vi "外观 2.vi"(0 "Data In":T5 caption="数据输入" format="%04x", 2 "Display State In":T3 caption="显示状态输入", 3 "Container State":T4 caption="容器状态") -> (6 "Data Out":T5 caption="数据输出" format="%04x", 7 "Display State Out":T3 caption="显示状态输出", 8 "Action":T2 caption="动作")   [LabVIEW 2016, in "总磷氨氮调试.xctl"]
uses:
  <vilib>/_xctls/Container State.ctl
  <vilib>/_xctls/Action.ctl
  <vilib>/_xctls/XControlSupport.lvlib
panel:
  out "选项卡控件":enum32{"选项卡 1", "选项卡 2"}(tab)
  in  "V9-2":bool
  in  "V9-1":bool
  in  "阀口选择":T1(radio)
  in  "阀口":enum32{"未选择", "V1开", "V1关", "V2开", "V2关"}(radio)
  in  "蠕动泵":enum32{"未选择", "P1", "P2"}(radio)
  in  "灯":enum32{"未选择", "520", "660", "加热恒温", "氙灯/紫灯"}(radio)
  in  "ADC值":enum32{"未选择", "ADC0", "降温温度", "消解温度", "光谱/ADC1"}(radio)
  in  "总磷总氮启动项目输入":enum32{"功能1", "功能2"}(ring)
  in  "功能选择":enum32{"等待", "复位", "注入", "注出"}(radio)=enum."注入"
  in  "数值":i16=4000
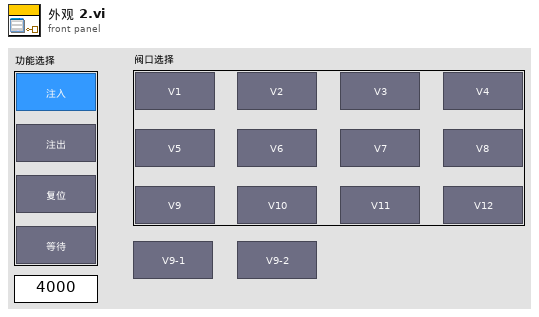
[diagram p1: front panel]
types:
  T1 = enum32{"未选择", "V1", "V2", "V3", "V4", "V5", "V6", "V7", "V8", "V9", "V10", "V11", "V12"}
  T2 = typedef "XControlSupport.lvlib/Action.ctl" = cluster{"Data Changed?":bool, "State Changed?":bool, "Action Name":string}
  T3 = typedef "总磷氨氮调试.xctl/状态 2.ctl" = cluster{"Numeric":dbl}
  T4 = typedef "XControlSupport.lvlib/Container State.ctl" = cluster{"Indicator?":bool, "Run Mode?":bool, " Refnum":refnum<vi>}
  T5 = typedef "总磷氨氮调试.xctl/数据 2.ctl" = u16[]
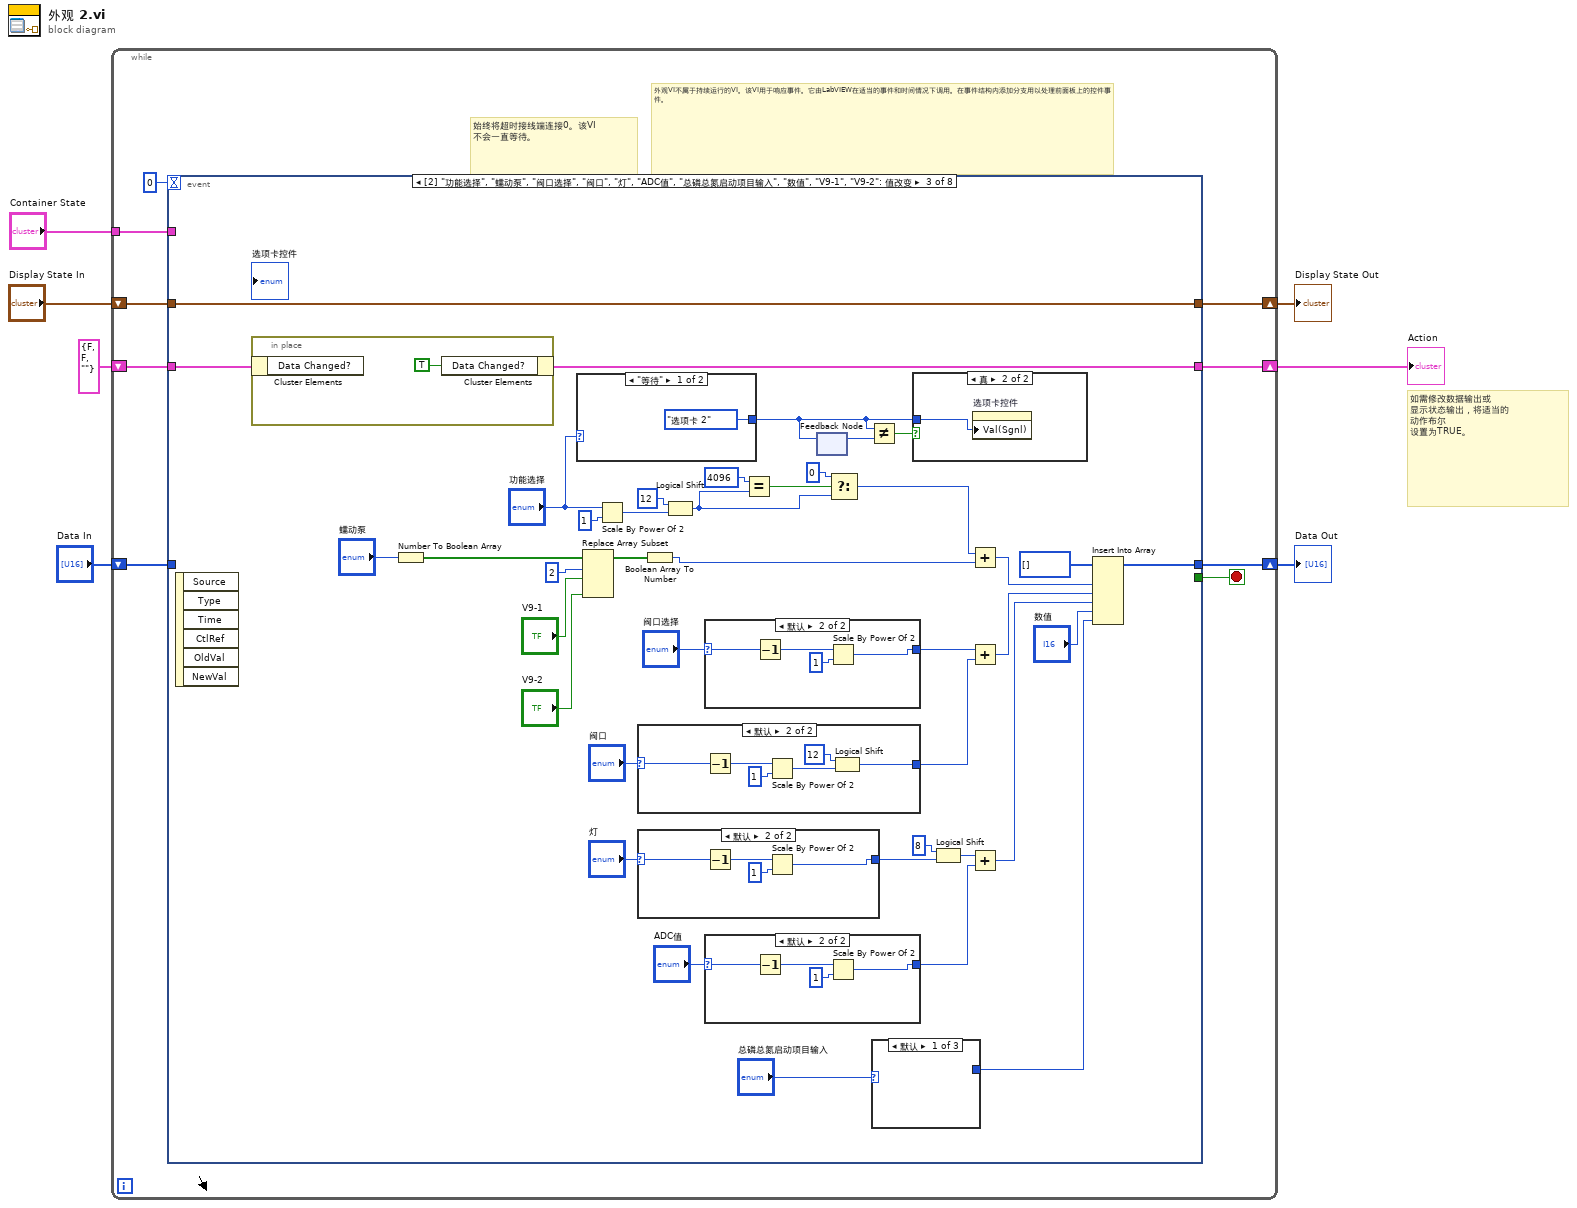
[diagram p0: block diagram]
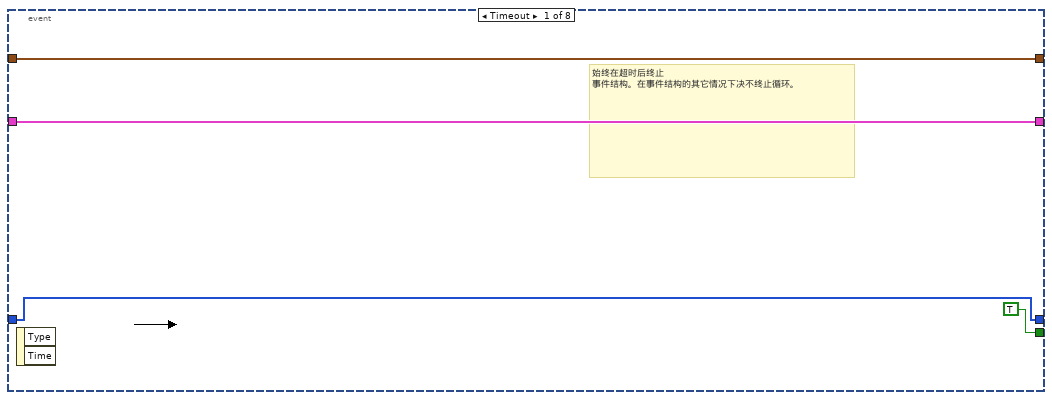
[diagram p2: hidden frame]
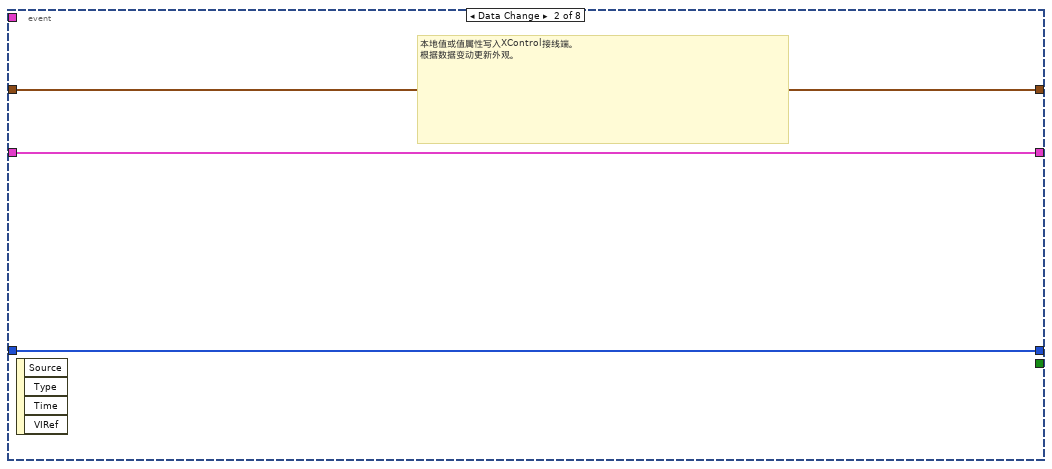
[diagram p3: hidden frame]
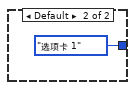
[diagram p5: hidden frame]
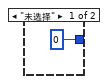
[diagram p6: hidden frame]
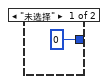
[diagram p7: hidden frame]
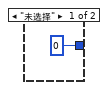
[diagram p8: hidden frame]
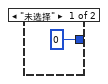
[diagram p9: hidden frame]
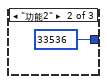
[diagram p10: hidden frame]
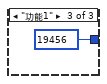
[diagram p11: hidden frame]
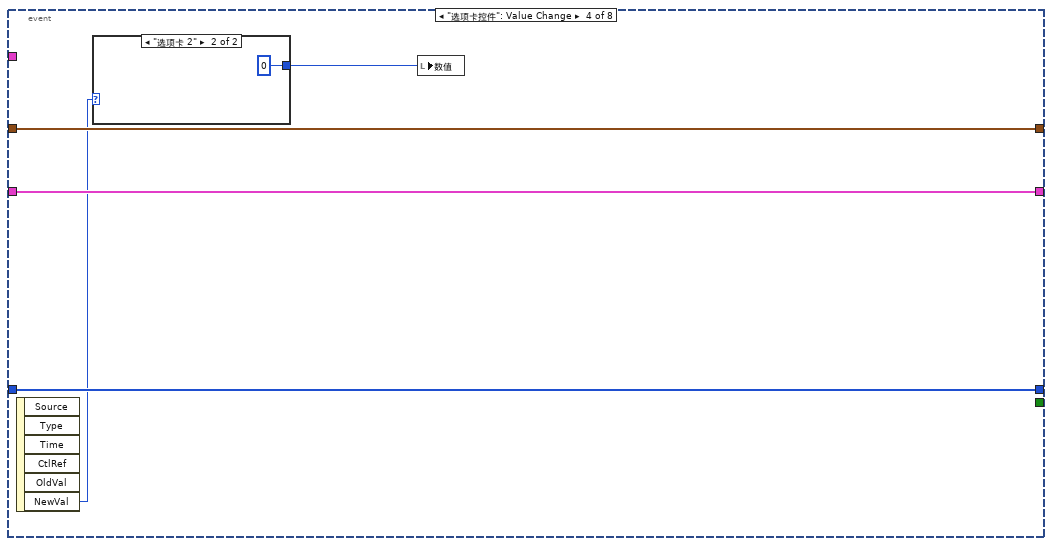
[diagram p12: hidden frame]
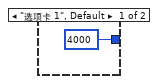
[diagram p13: hidden frame]
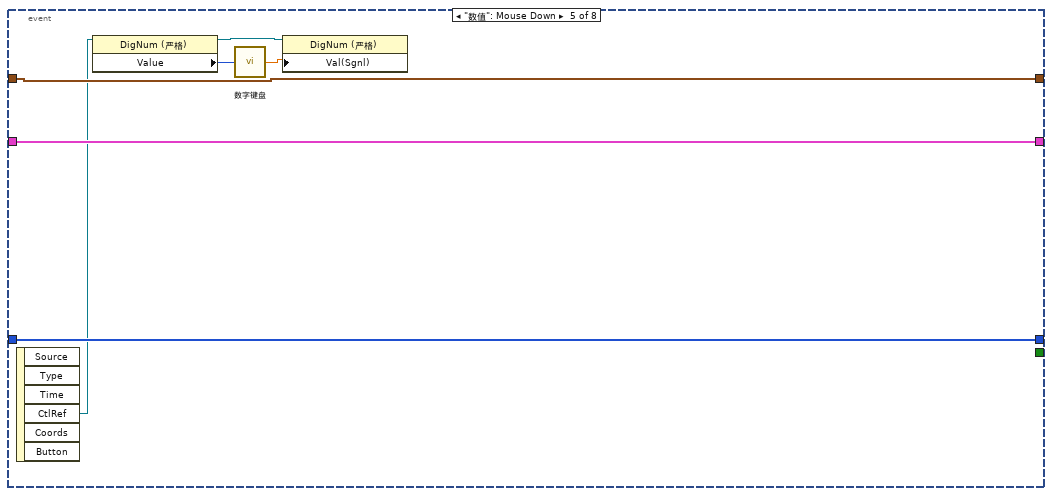
[diagram p14: hidden frame]
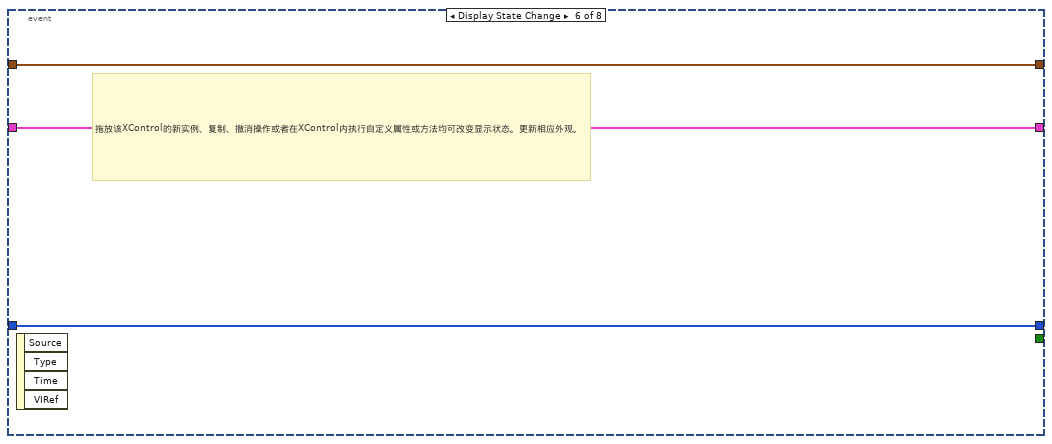
[diagram p15: hidden frame]
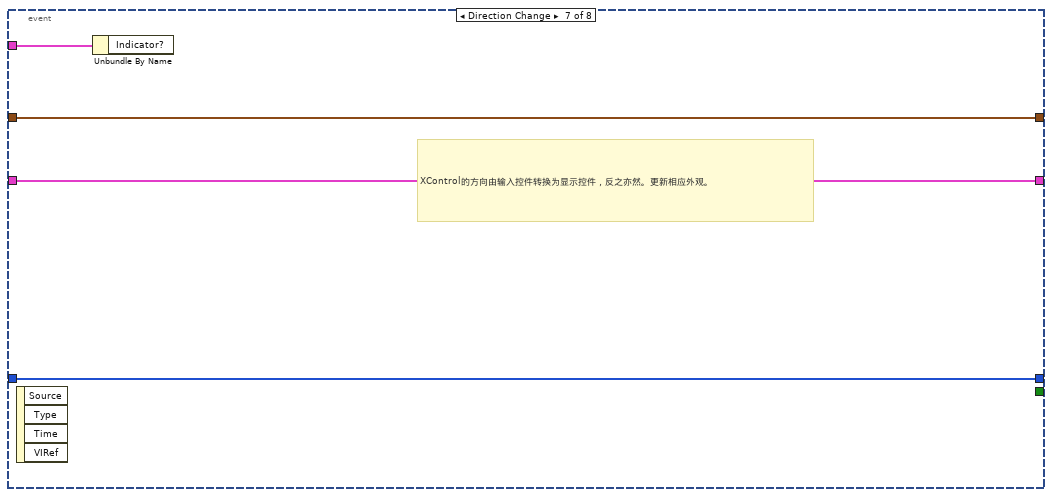
[diagram p16: hidden frame]
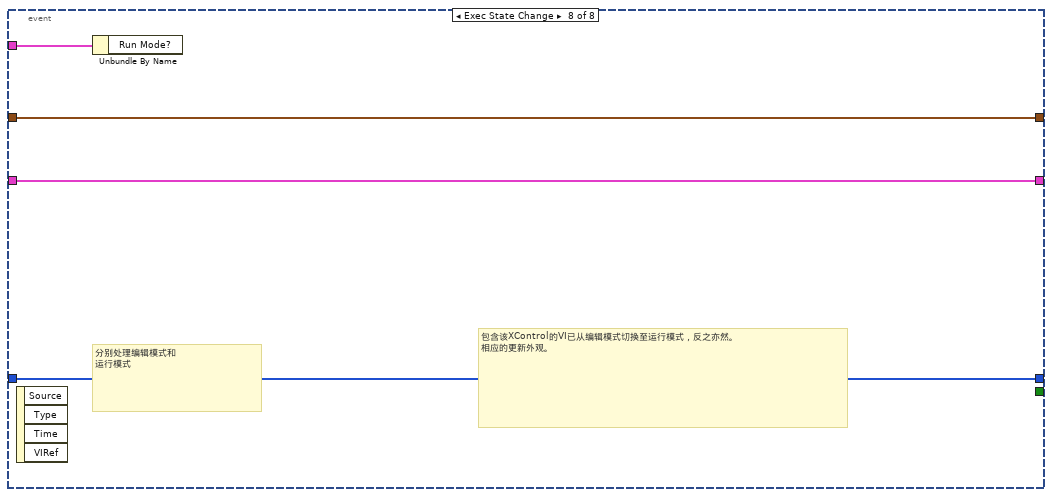
[diagram p17: hidden frame]
diagram:
  # "如需修改数据输出或\n显示状态输出，将适当的\n动作布尔\n设置为TRUE。"
  n1 = while {
    shift-right: [w15] -> w4
    shift-left: "Display State In" -> [w16]
    tunnel: "Container State" -> [w12]
    shift-right: [w10] -> w7
    shift-left: "Data In" -> [w11]
    shift-right: [w8] -> w2
    shift-left: T2 {"Data Changed?"=FALSE, "State Changed?"=FALSE, "Action Name"=""} ("Action") -> [w9]
    stop <- w14 stop-if-true
    # "外观VI不属于持续运行的VI。该VI用于响应事件。它由LabVIEW在适当的事件和时间情况下调用。在事件结构内添加分支用以处理前面板上的控件事件。"
    # "始终将超时接线端连接0。该VI\n不会一直等待。"
    n2 = event shown="[2] \"功能选择\", \"蠕动泵\", \"阀口选择\", \"阀口\", \"灯\", \"ADC值\", \"总磷总氮启动项目输入\", \"数值\", \"V9-1\", \"V9-2\": 值改变" {
      selector: _ -> [_ _ _ _ _ _ _ _]
      dyn-events: _ -> [_ _ _ _ _ _ _ _]
      timeout: 0 -> [_ _ _ _ _ _ _ _]
      tunnel: w16 -> [w18 w22 w63 w96 w105 w108 w111 w115]
      tunnel: [w18 w22 w63 w96 w105 w108 w111 w115] -> w15
      tunnel: [TRUE _ _ _ _ _ _ _] -> w14
      tunnel: w12 -> [_ _ _ _ _ _ w112 w116]
      tunnel: w11 -> [w17 w23 _ w95 w104 w107 w110 w114]
      tunnel: [w17 w23 w34 w95 w104 w107 w110 w114] -> w10
      tunnel: [w19 w21 w61 w94 w103 w106 w109 w113] -> w8
      tunnel: w9 -> [w19 w21 w62 w94 w103 w106 w109 w113]
      event Timeout {
        # "始终在超时后终止\n事件结构。在事件结构的其它情况下决不终止循环。"
        n3 = event-data() -> ()  [unwired: 1 in, 2 out]
      }
      event Data Change {
        # "本地值或值属性写入XControl接线端。\n根据数据变动更新外观。"
        n4 = event-data() -> ()  [unwired: 1 in, 4 out]
      }
      event "功能选择", "蠕动泵", "阀口选择", "阀口", "灯", "ADC值", "总磷总氮启动项目输入", "数值", "V9-1", "V9-2": Value Change {
        n5 = event-data() -> ()  [unwired: 1 in, 6 out]
        n6 = in-place {
          n7 = in-place-cluster #1(w62) -> ()  [unwired: 1 out]
          n8 = in-place-cluster #1("Data Changed?"=TRUE) -> (w61:T2)
        }
        n9 = Number To Boolean Array(number="蠕动泵") -> (Boolean array=w32:bool[])
        n10 = case shown="\"等待\"" "功能选择" {
          tunnel: [enum32{"选项卡 1", "选项卡 2"}."选项卡 2" ("选项卡控件") enum32{"选项卡 1", "选项卡 2"}."选项卡 1" ("选项卡控件")] -> w25
          frame "等待" {
          }
          frame Default {
          }
        }
        n11 = Replace Array Subset(array=w32, new element #1="V9-1", index #1=2 ("索引"), new element #2="V9-2") -> (w28:bool[])  [unwired: 1 in]
        n12 = Scale By Power Of 2(n="功能选择", x=i16 1 ("y")) -> (x*2^n=w46:i16)
        n13 = case shown="默认" "阀口" {
          selector: "阀口" -> [_ w82]
          tunnel: [i16 0 ("y") w78] -> w44
          frame "未选择" {
          }
          frame Default {
            n14 = Decrement(x=w82) -> (x-1=w83:enum32{"未选择", "V1开", "V1关", "V2开", "V2关"})
            n15 = Scale By Power Of 2(n=w83, x=i16 1 ("y")) -> (x*2^n=w80:i16)
            n16 = Logical Shift(y=i16 12, x=w80) -> (x << y=w78:i16)
          }
        }
        n17 = case shown="默认" "灯" {
          selector: "灯" -> [_ w74]
          tunnel: [i16 0 ("y") w76] -> w40
          frame "未选择" {
          }
          frame Default {
            n18 = Decrement(x=w74) -> (x-1=w75:enum32{"未选择", "520", "660", "加热恒温", "氙灯/紫灯"})
            n19 = Scale By Power Of 2(n=w75, x=i16 1 ("y")) -> (x*2^n=w76:i16)
          }
        }
        n20 = Boolean Array To Number(Boolean array=w28) -> (number=w24:u32)
        n21 = Logical Shift(y=i16 12, x=w46) -> (x << y=w52:i16)
        n22 = case shown="默认" "阀口选择" {
          selector: "阀口选择" -> [_ w86]
          tunnel: [i16 0 ("y") w88] -> w45
          frame "未选择" {
          }
          frame Default {
            n23 = Decrement(x=w86) -> (x-1=w87:T1)
            n24 = Scale By Power Of 2(n=w87, x=i16 1 ("y")) -> (x*2^n=w88:i16)
          }
        }
        n25 = case shown="默认" "ADC值" {
          selector: "ADC值" -> [_ w69]
          tunnel: [i16 0 ("y") w71] -> w39
          frame "未选择" {
          }
          frame Default {
            n26 = Decrement(x=w69) -> (x-1=w70:enum32{"未选择", "ADC0", "降温温度", "消解温度", "光谱/ADC1"})
            n27 = Scale By Power Of 2(n=w70, x=i16 1 ("y")) -> (x*2^n=w71:i16)
          }
        }
        n28 = Equal?(x=u32 4096 ("t"), y=w52) -> (x = y?=w60:bool)
        n29 = feedback-in #2(w25) -> ()
        n30 = feedback #2() -> (w27:enum32{"选项卡 1", "选项卡 2"})  [unwired: 1 in]
        n31 = Select(t=u32 0, s=w60, f=w52) -> (s? t:f=w50:u32)
        n32 = Not Equal?(x=w25, y=w27) -> (x != y?=w26:bool)
        n33 = case shown="默认" "总磷总氮启动项目输入" {
          tunnel: [_ 33536 19456] -> w48
          frame Default {
          }
          frame "功能2" {
          }
          frame "功能1" {
          }
        }
        n34 = case shown="真" w26 {
          tunnel: w25 -> [_ w64]
          frame False {
          }
          frame True {
            n35 = property on="选项卡控件" class="TabCtl (严格)"("Val(Sgnl)"=w64) -> ()  [unwired: 2 in, 2 out]
          }
        }
        n36 = Logical Shift(y=i16 8, x=w40) -> (x << y=w58:i16)
        n37 = Add(x=w50, y=w24) -> (x+y=w55:u32)
        n38 = Add(x=w45, y=w44) -> (x+y=w43:i16)
        n39 = Add(x=w58, y=w39) -> (x+y=w54:i16)
        n40 = Insert Into Array(array=u16[] [] ("数组"), new element #1=w55, new element #2=w43, new element #3=w54, new element #4="数值", new element #5=w48) -> (w34:u16[])  [unwired: 1 in]
      }
      event "选项卡控件": Value Change {
        n41 = event-data() -> ("NewVal"=w93:enum32{"选项卡 1", "选项卡 2"})  [unwired: 1 in, 5 out]
        n42 = case shown="\"选项卡 2\"" w93 {
          tunnel: [i16 4000 ("数值") i16 0 ("数值")] -> w92
          frame "选项卡 1", Default {
          }
          frame "选项卡 2" {
          }
        }
        n43 = local write "数值"(w92) -> ()
      }
      event "数值": Mouse Down {
        n44 = event-data() -> ("CtlRef"=w102:refnum<vi>)  [unwired: 1 in, 5 out]
        n45 = property class="DigNum (严格)"(reference=w102) -> (reference out=w101:refnum<vi>, "Value"=w100:i16)  [unwired: 1 in, 1 out]
        n46 = call "数字键盘.vi"("OldNumber"=w100) -> ("NewNumber"=w99:sgl)
        n47 = property class="DigNum (严格)"(reference=w101, "Val(Sgnl)"=w99) -> ()  [unwired: 1 in, 2 out]
      }
      event Display State Change {
        # "拖放该XControl的新实例、复制、撤消操作或者在XControl内执行自定义属性或方法均可改变显示状态。更新相应外观。"
        n48 = event-data() -> ()  [unwired: 1 in, 4 out]
      }
      event Direction Change {
        # "XControl的方向由输入控件转换为显示控件，反之亦然。更新相应外观。"
        n49 = event-data() -> ()  [unwired: 1 in, 4 out]
        n50 = Unbundle By Name(w112) -> ()  [unwired: 1 out]
      }
      event Exec State Change {
        # "包含该XControl的VI已从编辑模式切换至运行模式，反之亦然。\n相应的更新外观。"
        # "分别处理编辑模式和\n运行模式"
        n51 = event-data() -> ()  [unwired: 1 in, 4 out]
        n52 = Unbundle By Name(w116) -> ()  [unwired: 1 out]
      }
    }
  }
  "Display State Out" <- w4
  "Data Out" <- w7
  "Action" <- w2
